vi "Registered Objects.vi"(7 "Action":T1(ring), 8 "error in (no error)":errorcluster, 11 "Object Name":string) -> (0 "error out":errorcluster, 3 "Is Registered":bool=TRUE)   [LabVIEW 2020, in "Provider.lvlib"]
uses:
  Provider.lvlib
  <vilib>/ErrorRing/Error Ring.xnode
  <vilib>/Utility/error.llb/Error Cluster From Error Code.vi
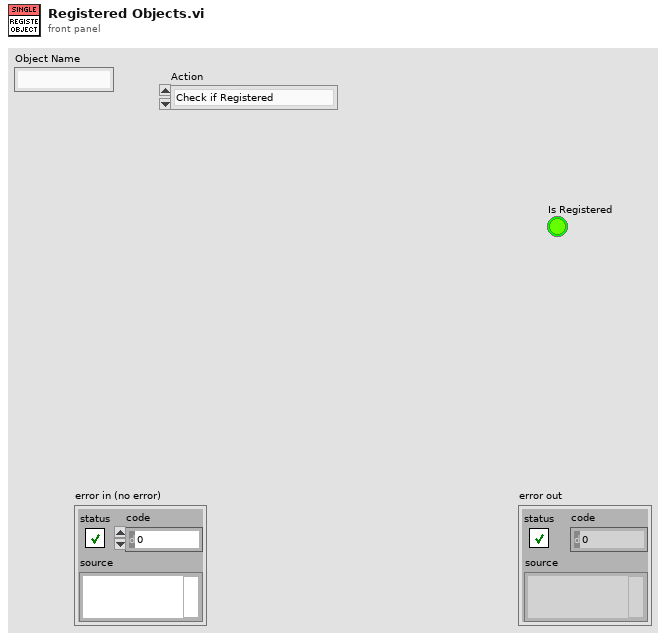
[diagram p1: front panel]
types:
  T1 = enum16{"Check if Registered", "Register Object", "Deregister Object", "Init"}
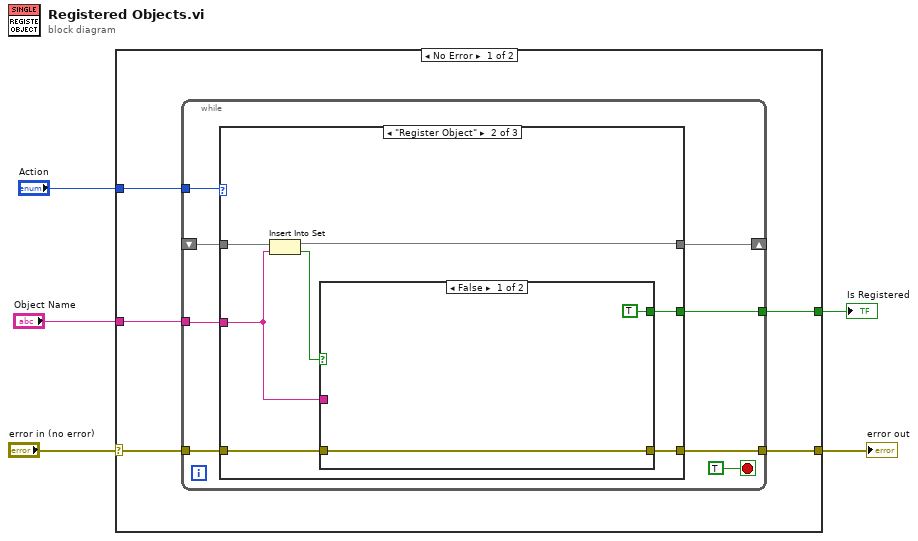
[diagram p0: block diagram]
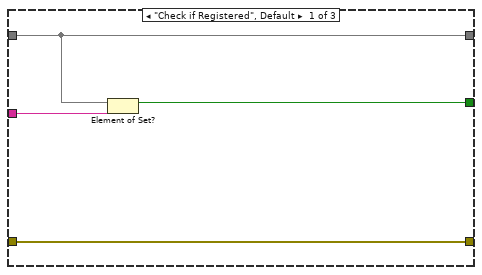
[diagram p2: hidden frame]
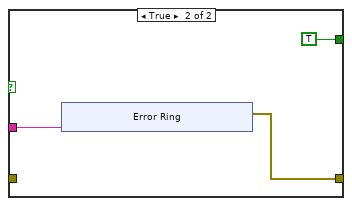
[diagram p3: hidden frame]
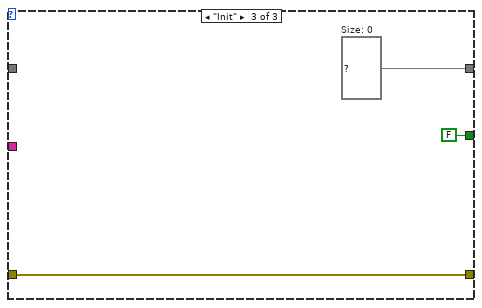
[diagram p4: hidden frame]
diagram:
  n1 = case shown="No Error" "error in (no error)" {
    selector: "error in (no error)" -> [w9 w45]
    tunnel: [w10 w45] -> w4
    tunnel: "Action" -> [w8 _]
    tunnel: "Object Name" -> [w7 _]
    tunnel: [w6 _] -> w1
    frame No Error {
      n2 = while {
        tunnel: [w18] -> w10
        tunnel: w9 -> [w17]
        tunnel: w8 -> [w15]
        tunnel: w7 -> [w14]
        shift-right: [w13] -> _
        shift-left: _ -> [w12]
        tunnel: [w11] -> w6
        stop <- TRUE stop-if-true
        n3 = case shown="\"Register Object\"" w15 {
          tunnel: [w22 w24 w44] -> w18
          tunnel: w17 -> [w22 w25 w44]
          tunnel: w14 -> [w21 w26 _]
          tunnel: [w20 w28 w43] -> w13
          tunnel: w12 -> [w20 w29 _]
          tunnel: [w19 w23 FALSE ("found?")] -> w11
          frame "Check if Registered", Default {
            n4 = Element of Set?(10:w21, 11:w20) -> (3:w19:bool)
          }
          frame "Register Object" {
            n5 = Insert Into Set(10:w26, 11:w29) -> (2:w27:bool, 3:w28:set{string})
            n6 = case shown="False" w27 {
              tunnel: w26 -> [_ w34]
              tunnel: w25 -> [w31 _]
              tunnel: [w31 w33] -> w24
              tunnel: [TRUE TRUE] -> w23
              frame False {
              }
              frame True {
                n7 = xnode "Error Ring"("parameter 0"=w34) -> ("error out"=w33:errorcluster)
              }
            }
          }
          frame "Init" {
            w43 = set{string} {}  # Size: 0
          }
        }
      }
    }
    frame Error {
    }
  }
  "error out" <- w4
  "Is Registered" <- w1
